vi "onTestDiscovery.vi"(8 "error in (no error)":errorcluster, 11 "DMC Folder Test Runner in":refnum<class "DMC Folder Test Runner.lvclass">) -> (0 "error out":errorcluster, 2 "Tests VIs":path[](array[path]), 3 "DMC Folder Test Runner out":refnum<class "DMC Folder Test Runner.lvclass">)   [LabVIEW 2023, in "DMC Folder Test Runner.lvclass"]
uses:
  DMC Folder Test Runner.lvclass
  C:/Program Files/National Instruments/LabVIEW 2023/vi.lib/addons/_JKI Toolkits/Caraya/classes/Test Runner/Test Runner.lvclass
  DMC Folder Test Runner.lvclass/DMC Folder Test Runner.ctl
  <vilib>/addons/_JKI Toolkits/Caraya/classes/Test Runner.Folder/Test Runner.Folder.lvclass
  <vilib>/addons/_JKI Toolkits/Caraya/classes/Test Runner/Test Runner.lvclass
  C:/Program Files/National Instruments/LabVIEW 2023/vi.lib/addons/_JKI Toolkits/Caraya/classes/Test Runner.Folder/Test Runner.Folder.lvclass
  C:/projects/DMC/GitHub/DMC CLI Caraya/Source/DMC Folder Test Runner/DMC Folder Test Runner.lvclass
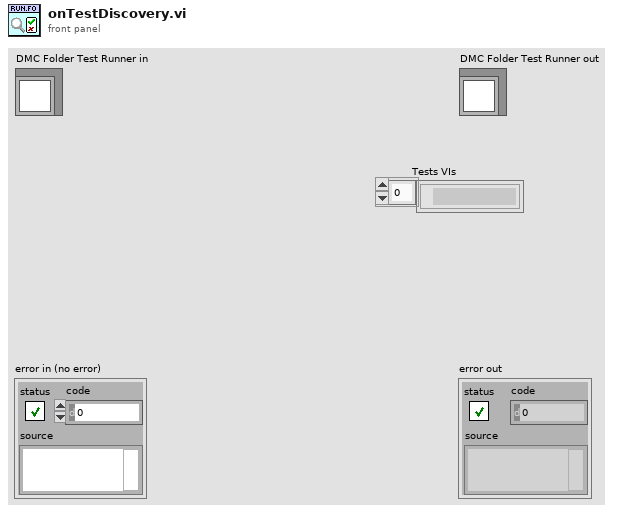
[diagram p1: front panel]
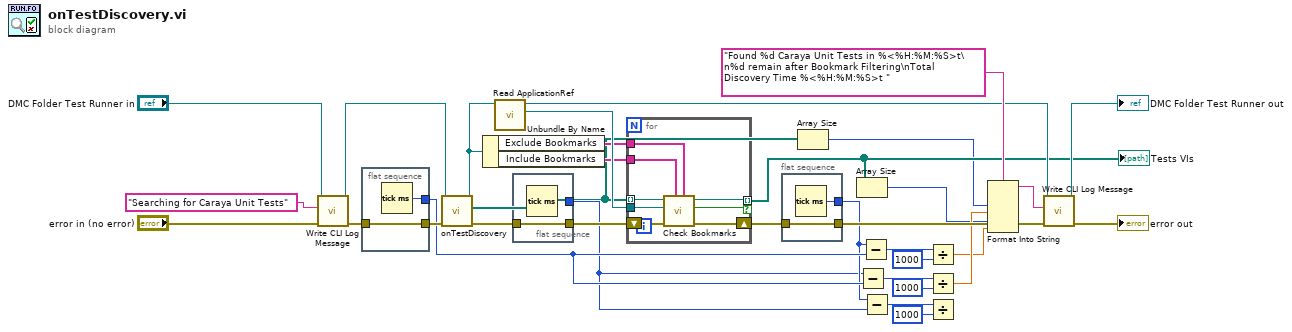
[diagram p0: block diagram]
diagram:
  n1 = call "Write CLI Log Message.vi"("error in (no error)"="error in (no error)", "Message"="Searching for Caraya Unit Tests", "DMC Folder Test Runner in"="DMC Folder Test Runner in") -> ("error out"=w29:errorcluster, "DMC Folder Test Runner out"=w33:refnum<class "DMC Folder Test Runner.lvclass">)  [unwired: 7 in]
  n2 = flat-sequence {
    tunnel: [w36] -> w30
    tunnel: w29 -> [w36]
    tunnel: [w35] -> w12
    frame #0 {
      n3 = Tick Count (ms)() -> (millisecond timer value=w35:u32)
    }
  }
  n4 = call-parent "onTestDiscovery.vi"("error in (no error)"=w30, "Test Runner.Folder in"=w33) -> ("error out"=w14:errorcluster, "Tests VIs"=w4:path[], "Test Runner.Folder out"=w19:refnum<class "DMC Folder Test Runner.lvclass">)  [unwired: 7 in]
  n5 = Unbundle By Name(w19) -> ("Exclude Bookmarks"=w18:string[], "Include Bookmarks"=w17:string[])
  n6 = call <vilib>:"Read ApplicationRef.vi"("Test Runner in"=w19) -> ("Application"=w20:refnum<vi>, "Test Runner out"=w21:refnum<class "DMC Folder Test Runner.lvclass">)  [unwired: 8 in, 1 out]
  n7 = flat-sequence {
    tunnel: [w38] -> w10
    tunnel: [w37] -> w13
    tunnel: w14 -> [w37]
    frame #0 {
      n8 = Tick Count (ms)() -> (millisecond timer value=w38:u32)
    }
  }
  n9 = for {
    tunnel: w4 -> [w45] mode=indexing
    shift-right: [w41] -> w15
    shift-left: w13 -> [w46]
    tunnel: w20 -> [w44]
    tunnel: w18 -> [w43]
    tunnel: w17 -> [w42]
    tunnel: [w40] -> w16 mode=indexing if=w39
    n10 = call "Check Bookmarks.vi"("Exclude Bookmarks"=w43, "Include Bookmarks"=w42, "error in (no error)"=w46, "App Ref"=w44, "VI Path"=w45) -> ("error out"=w41:errorcluster, "Check If Unit Test?"=w39:bool, "VI Path dup"=w40:path)  [unwired: 4 in]
  }
  "Tests VIs" <- w16
  n11 = flat-sequence {
    tunnel: [w48] -> w11
    tunnel: [w47] -> w25
    tunnel: w15 -> [w47]
    frame #0 {
      n12 = Tick Count (ms)() -> (millisecond timer value=w48:u32)
    }
  }
  n13 = Array Size(array=w4) -> (size(s)=w3:i32)
  n14 = Array Size(array=w16) -> (size(s)=w2:i32)
  n15 = Subtract(x=w10, y=w12) -> (x-y=w6:u32)
  n16 = Subtract(x=w11, y=w12) -> (x-y=w26:u32)
  n17 = Subtract(x=w11, y=w10) -> (x-y=w7:u32)
  n18 = Divide(x=w26, y=u32 1000) -> (x/y=w1:dbl)
  n19 = Divide(x=w6, y=u32 1000) -> (x/y=w5:dbl)
  n20 = Divide(x=w7, y=u32 1000) -> ()  [unwired: 1 out]
  n21 = Format Into String(format string="Found %d Caraya Unit Tests in %<%H:%M:%S>t\n%d remain after Bookmark Filtering\nTotal Discovery Time %<%H:%M:%S>t ", w3, w5, w2, w1) -> (resulting string=w22:string)  [unwired: 2 in, 1 out]
  n22 = call "Write CLI Log Message.vi"("error in (no error)"=w25, "Message"=w22, "DMC Folder Test Runner in"=w21) -> ("error out"=→"error out":errorcluster, "DMC Folder Test Runner out"=→"DMC Folder Test Runner out":refnum<class "DMC Folder Test Runner.lvclass">)  [unwired: 7 in]
